vi "Update Map.vi"(7 "Moved?":bool, 9 "New Position":T1, 10 "Old Position":T1, 11 "Map in":i32[][](array[numeric])) -> (3 "Map":i32[][](array[numeric]))   [LabVIEW 2015, in "Border.lvclass"]
uses:
  Border.lvclass
  Common/Position.ctl
  Common/Common.lvlib
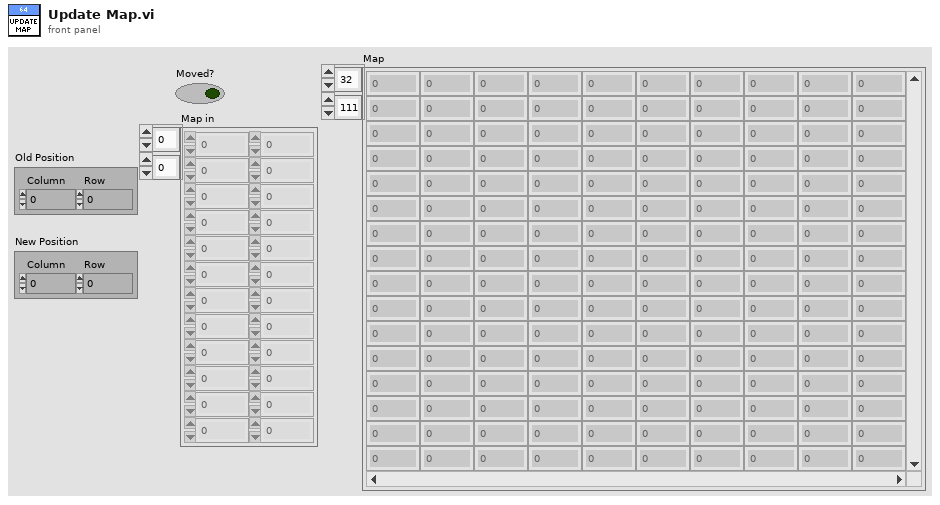
[diagram p1: front panel]
types:
  T1 = typedef "Common.lvlib/Position.ctl" = cluster{"Column":i32, "Row":i32}
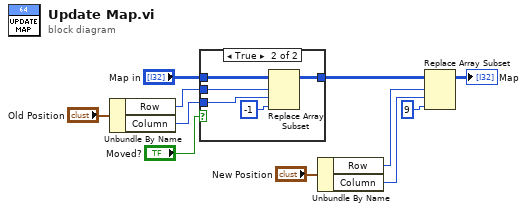
[diagram p0: block diagram]
diagram:
  n1 = Unbundle By Name("Old Position") -> ("Row"=w10:i32, "Column"=w9:i32)
  n2 = case shown="True" "Moved?" {
    tunnel: "Map in" -> [w12 w17]
    tunnel: [w12 w16] -> w3
    tunnel: w10 -> [_ w15]
    tunnel: w9 -> [_ w14]
    frame False {
    }
    frame True {
      n3 = Replace Array Subset(array=w17, new element=-1 ("new element/subarray"), index (row)=w15, index (col)=w14) -> (w16:i32[][])
    }
  }
  n4 = Unbundle By Name("New Position") -> ("Row"=w7:i32, "Column"=w6:i32)
  n5 = Replace Array Subset(array=w3, new element=9 ("new element/subarray"), index (row)=w7, index (col)=w6) -> (→"Map":i32[][])
